vi "RelayAction to RelayPosition.vi"(10 "action":T2=21 caption="relay action" items=["CloseRelay"=21, "OpenRelay"=20]) -> (2 "position":T1=11 items=["Open"=10, "Closed"=11])   [LabVIEW 2015, in "SLSC Switch.lvlib" / "slscsl.lvclass"]
uses:
  slscsl.lvclass
  RelayAction.ctl
  RelayPosition.ctl
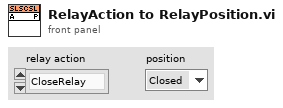
[diagram p1: front panel]
types:
  T1 = typedef "SLSC Switch.lvlib/slscsl.lvclass/RelayPosition.ctl" = i32
  T2 = typedef "SLSC Switch.lvlib/slscsl.lvclass/RelayAction.ctl" = u32
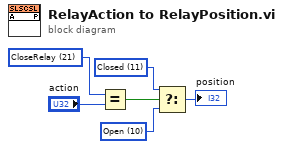
[diagram p0: block diagram]
diagram:
  w1 = T2 21 items=["CloseRelay"=21, "OpenRelay"=20] ("RelayAction")
  w4 = T1 10 items=["Open"=10, "Closed"=11] ("f")
  w5 = T1 11 items=["Open"=10, "Closed"=11] ("x")
  n1 = Equal?(x=w1, y="action") -> (x = y?=w6:bool)
  n2 = Select(t=w5, s=w6, f=w4) -> (s? t:f=→"position":T1)
